vi "Pickup Tool.vi"(8 "error in":errorcluster, 10 "Tool":string, 11 "Gantry in":refnum<class "Gantry.lvclass">) -> (0 "error out":errorcluster, 3 "Gantry out":refnum<class "Gantry.lvclass">)   [LabVIEW 2017, in "Gantry.lvclass"]
uses:
  Gantry.lvclass
  FlexWorktable/FlexWorktable.lvclass
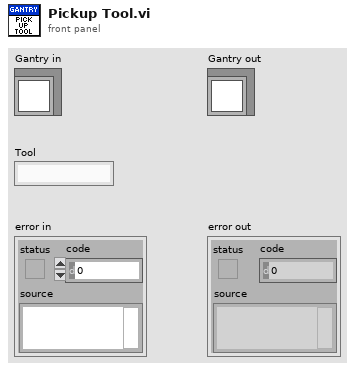
[diagram p1: front panel]
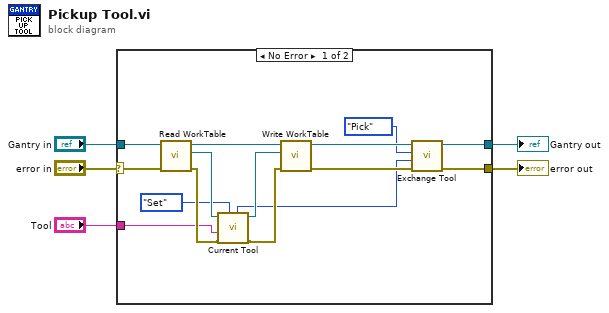
[diagram p0: block diagram]
diagram:
  n1 = case shown="No Error" "error in" {
    selector: "error in" -> [w19 w22]
    tunnel: [w13 w22] -> w4
    tunnel: [w14 w21] -> w2
    tunnel: "Gantry in" -> [w20 w21]
    tunnel: "Tool" -> [w8 _]
    frame No Error {
      n2 = call-dynamic "Read WorkTable.vi"("error in"=w19, "Gantry Class in"=w20) -> ("error out"=w10:errorcluster, "Worktable"=w12:refnum<class "FlexWorktable.lvclass">, "Gantry Class out"=w18:refnum<class "Gantry.lvclass">)  [unwired: 7 in]
      n3 = call-dynamic "Current Tool.vi"("Get/Set"=enum16{"Get", "Set"}."Set", "error in (no error)"=w10, "Tool in"=w8, "FlexWorktable in"=w12) -> ("error out"=w9:errorcluster, "FlexWorktable out"=w11:refnum<class "FlexWorktable.lvclass">, "Rack Position"=w6:i32)  [unwired: 4 in, 1 out]
      n4 = call-dynamic "Write WorkTable.vi"("error in (no error)"=w9, "FlexWorktable"=w11, "Gantry Class in"=w18) -> ("error out"=w16:errorcluster, "Gantry Class out"=w17:refnum<class "Gantry.lvclass">)  [unwired: 7 in]
      n5 = call-dynamic "Exchange Tool.vi"("error in"=w16, "Tool Position"=w6, "Place/Pick"=enum16{"Place", "Pick"}."Pick", "Gantry in"=w17) -> ("error out"=w13:errorcluster, "Gantry out"=w14:refnum<class "Gantry.lvclass">)  [unwired: 6 in]
    }
    frame Error {
    }
  }
  "error out" <- w4
  "Gantry out" <- w2
